vi "Write NumberOfTactics.vi"(8 "error in (no error)":errorcluster, 10 "NumberOfTactics":dbl=2.0, 11 "ABCFirstKickerRole in":refnum<class "ABCFirstKickerRole.lvclass">) -> (0 "error out":errorcluster, 3 "ABCFirstKickerRole out":refnum<class "ABCFirstKickerRole.lvclass">)   [LabVIEW 2023, in "ABCFirstKickerRole.lvclass"]
uses:
  ABCFirstKickerRole.lvclass
  ABCFirstKickerRole.lvclass/ABCFirstKickerRole.ctl
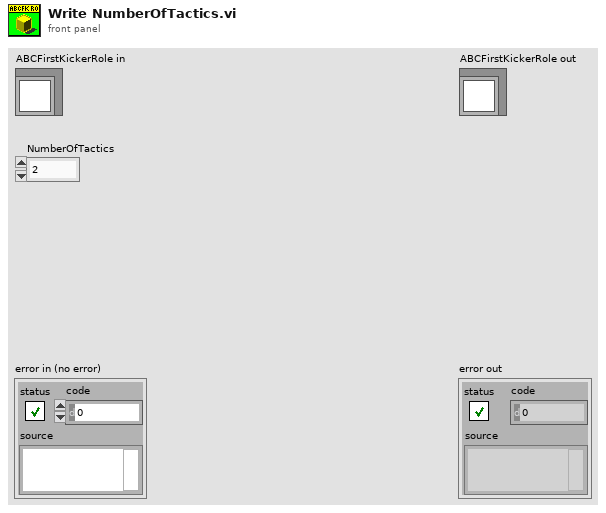
[diagram p1: front panel]
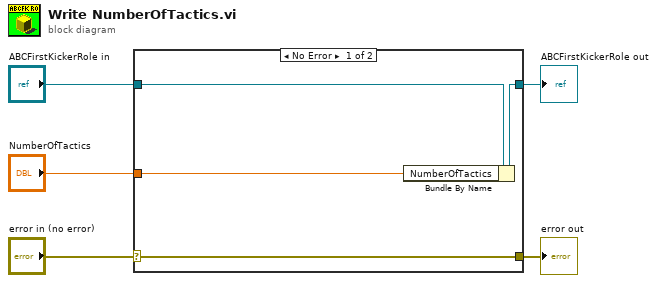
[diagram p0: block diagram]
diagram:
  n1 = case shown="No Error" "error in (no error)" {
    selector: "error in (no error)" -> [w9 w10]
    tunnel: [w9 w10] -> w4
    tunnel: [w7 w11] -> w2
    tunnel: "ABCFirstKickerRole in" -> [w8 w11]
    tunnel: "NumberOfTactics" -> [w6 _]
    frame No Error {
      n2 = Bundle By Name(cluster=w8, "NumberOfTactics"=w6) -> (w7:refnum<class "ABCFirstKickerRole.lvclass">)
    }
    frame Error {
    }
  }
  "error out" <- w4
  "ABCFirstKickerRole out" <- w2
